vi "RWA_File String.vi"(6 "Read(f) Write(t)":bool, 8 "Error":errorcluster, 9 "Section Name":string, 10 "File String":string, 11 "Anything":variant) -> (0 "Error Out":errorcluster, 1 "Data  Has Changed Out":bool, 2 "File String Out":string, 3 "Anything Out":variant, 5 "Message Out":string)   [LabVIEW 2020]
uses:
  MGI RWA Options Cluster.ctl
  <vilib>/Utility/Data Type/NI_Data Type.lvlib
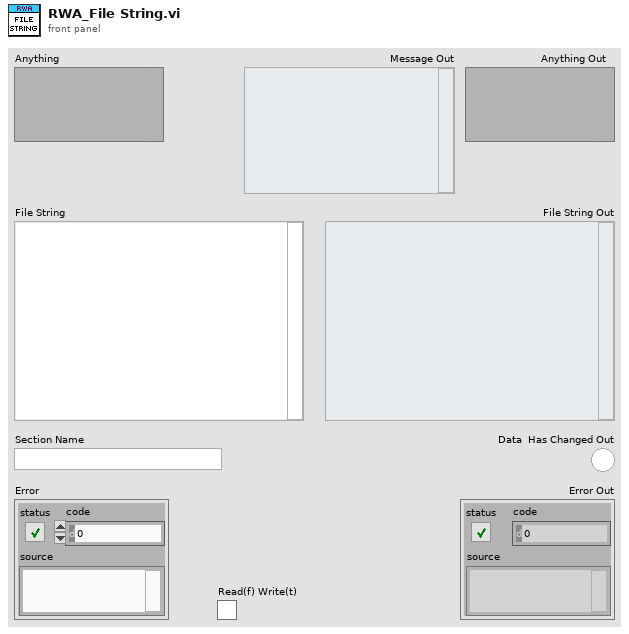
[diagram p1: front panel]
types:
  T1 = typedef "MGI RWA Options Cluster.ctl" = cluster{"TS Fmt":string, "Int Fmt":string, "Delimiter":string}
  T2 = typedef "NI_Data Type.lvlib/Type Definition Info.ctl" = cluster{"Name":string, "Timestamp":u32}
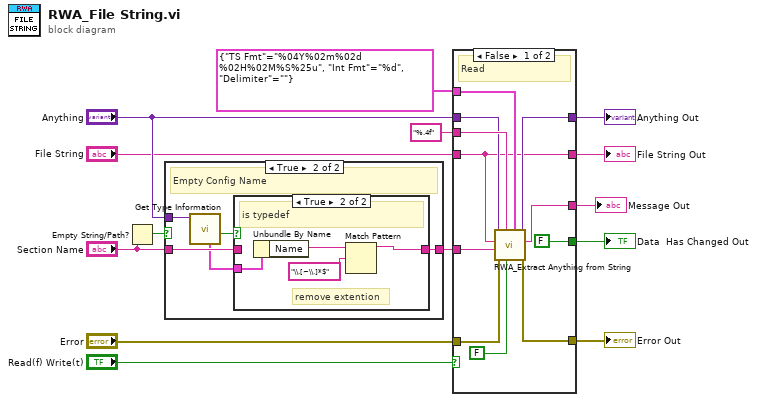
[diagram p0: block diagram]
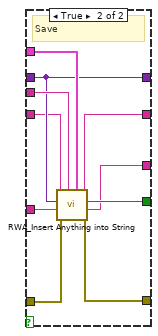
[diagram p4: hidden frame]
diagram:
  n1 = Empty String/Path?(string/path="Section Name") -> (empty?=w9:bool)
  n2 = case shown="True" w9 {
    tunnel: "Anything" -> [_ w20]
    tunnel: "Section Name" -> [w15 w18]
    tunnel: [w15 w16] -> w6
    frame False {
      # "Config Name provided"
    }
    frame True {
      # "Empty Config Name"
      n3 = call <vilib>:"Get Type Information.vi"("variant"=w20) -> ("type definition"=w19:bool, "type definition info"=w17:T2)  [unwired: 6 in, 3 out]
      n4 = case shown="True" w19 {
        tunnel: w18 -> [w21 _]
        tunnel: w17 -> [_ w25]
        tunnel: [w21 w22] -> w16
        frame False {
          # "Not a typedef"
        }
        frame True {
          # "remove extention"
          # "is typedef"
          n5 = Unbundle By Name(w25) -> ("Name"=w23:string)
          n6 = Match Pattern(string=w23, regular expression="\\.[~\\.]*$") -> (before substring=w22:string)  [unwired: 4 out]
        }
      }
    }
  }
  n7 = case shown="False" "Read(f) Write(t)" {
    tunnel: "Anything" -> [w29 w43]
    tunnel: "%.4f" ("Format String (%#_13g)") -> [w30 w46]
    tunnel: T1 {"TS Fmt"="%04Y%02m%02d %02H%02M%S%25u", "Int Fmt"="%d", "Delimiter"=""} ("Read/Write Options") -> [w36 w45]
    tunnel: w6 -> [w35 w44]
    tunnel: [w32 w39] -> w11
    tunnel: "Error" -> [w31 w41]
    tunnel: [w33 w43] -> w10
    tunnel: [FALSE ("Section Replaced? Out") w40] -> w5
    tunnel: "File String" -> [w28 w42]
    tunnel: [w28 w38] -> w2
    tunnel: [w26 w37] -> w1
    frame False {
      # "Read"
      n8 = call "RWA_Extract Anything from String.vi"("Read/Write Options (Version 1.x)"=w36, "Use Supplied (F: Use Default)"=FALSE, "Format String (%#_13g)"=w30, "Error"=w31, "Section Name"=w35, "File String"=w28, "Type Of Anything"=w29) -> ("Error Out"=w32:errorcluster, "Read Failures Out"=w26:string, "Anything Out"=w33:variant)  [unwired: 2 out]
    }
    frame True {
      # "Save"
      n9 = call "RWA_Insert Anything into String.vi"("Read/Write Options"=w45, "Format String (%#_13g)"=w46, "Error"=w41, "Section Name (Name Of \"Anything\")"=w44, "Anything"=w43, "File String"=w42) -> ("Error Out"=w39:errorcluster, "Write Warnings Out"=w37:string, "Section Replaced? Out"=w40:bool, "File String Out"=w38:string)  [unwired: 2 in]
    }
  }
  "Error Out" <- w11
  "Anything Out" <- w10
  "Data  Has Changed Out" <- w5
  "File String Out" <- w2
  "Message Out" <- w1
